vi "TCPwrite8bytes.vi"(8 "Error in":errorcluster, 10 "Cmd In":string, 11 "connection ID in":refnum<k5>) -> (0 "Error out":errorcluster, 3 "connection ID out":refnum<k5>)   [LabVIEW 2013]
panel:
  out "TCP receiving time":u32
  out "TCP time in":u32
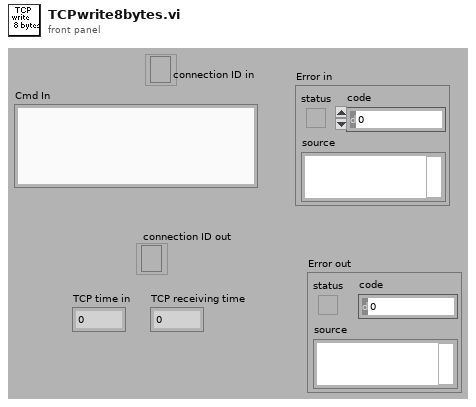
[diagram p1: front panel]
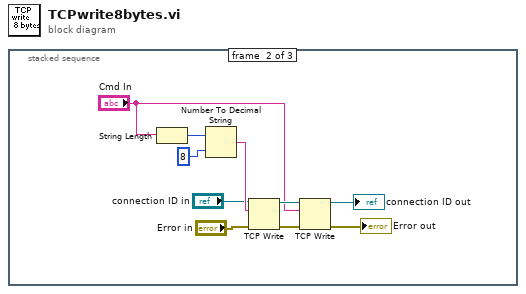
[diagram p0: block diagram]
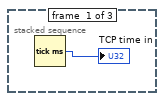
[diagram p2: hidden frame]
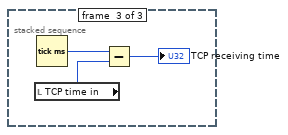
[diagram p3: hidden frame]
diagram:
  n1 = stacked-sequence {
    frame #0 {
      n2 = Tick Count (ms)() -> (millisecond timer value=→"TCP time in":u32)
    }
    frame #1 {
      n3 = String Length(string="Cmd In") -> (length=w9:i32)
      n4 = Number To Decimal String(number=w9, width (-)=i16 8) -> (decimal integer string=w11:string)
      n5 = TCP Write(connection ID="connection ID in", data in=w11, error in (no error)="Error in") -> (connection ID out=w8:refnum<k5>, error out=w7:errorcluster)  [unwired: 2 out]
      n6 = TCP Write(connection ID=w8, data in="Cmd In", error in (no error)=w7) -> (connection ID out=→"connection ID out":refnum<k5>, error out=→"Error out":errorcluster)  [unwired: 2 out]
    }
    frame #2 {
      n7 = local read "TCP time in"() -> (w12:u32)
      n8 = Tick Count (ms)() -> (millisecond timer value=w14:u32)
      n9 = Subtract(x=w14, y=w12) -> (x-y=→"TCP receiving time":u32)
    }
  }
